vi "Pre Launch Init.vi"(11 "Error Handler in":refnum<class "Error Handler.lvclass">) -> (0 "error out":errorcluster, 3 "Error Handler out":refnum<class "Error Handler.lvclass">)   [LabVIEW 2021, in "Error Handler.lvlib" / "Error Handler.lvclass"]
doc: "(<B>Filename</B>: Actor Framework.lvlib:Actor.lvclass:Pre Launch Init.vi)\n\nDefines behavior that occurs after the Launch Nested Actor method is invoked but before the actor's Actor Core method begins running.\n\nBy default, this method does nothing. A descendant class may override it to define behavior."
uses:
  Error Handler.lvclass
  Error Handler.lvclass/Error Handler.ctl
  Common/Common/Common.lvclass
  public types/response.ctl
  Error Handler.lvlib
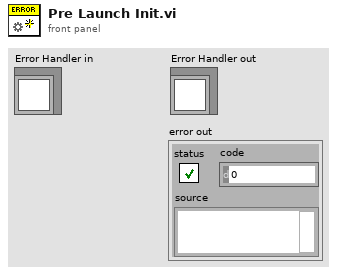
[diagram p1: front panel]
types:
  T1 = cluster{"status":bool, "code":i32, "source":string, "timestamp":dbl}
  T2 = typedef "Error Handler.lvlib/response.ctl" = enum16{"log", "log & popup", "log & exit", "log & popup & exit", "popup", "popup & exit", "exit", "ignore"}
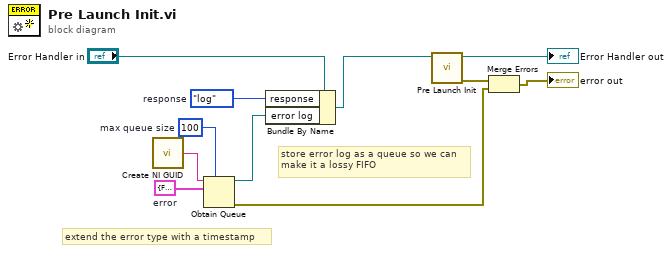
[diagram p0: block diagram]
diagram:
  w9 = T1 {"status"=FALSE, "code"=0, "source"="", "timestamp"=0.0}  # error
  w6 = response."log"  # response
  w8 = 100  # max queue size
  # "store error log as a queue so we can\nmake it a lossy FIFO"
  # "extend the error type with a timestamp"
  n1 = call <vilib>:"Create NI GUID.vi"() -> ("NI GUID"=w7:string)
  n2 = Obtain Queue(max queue size (-1, unlimited)=w8, name (unnamed)=w7, element data type=w9) -> (queue out=w1:refnum<queue>, error out=w2:errorcluster)  [unwired: 2 in, 1 out]
  n3 = Bundle By Name(cluster="Error Handler in", "response"=w6, "error log"=w1) -> (w4:refnum<class "Error Handler.lvclass">)
  n4 = call-parent "Pre Launch Init.vi"("Common in"=w4) -> ("error out"=w11:errorcluster, "Common out"=→"Error Handler out":refnum<class "Error Handler.lvclass">)  [unwired: 9 in]
  n5 = Merge Errors(w11, w2) -> (→"error out":errorcluster)
